vi "to table.vi"(8 "error in (no error)":errorcluster, 10 "variant":variant, 11 "Scaling editor node in":refnum<class "Scaling editor node.lvclass">) -> (0 "error out":errorcluster, 2 "table":string[][](array[string]), 3 "Scaling editor node out":refnum<class "Scaling editor node.lvclass">)   [LabVIEW 2013, in "Scaling editor node.lvclass"]
uses:
  Scaling editor node.lvclass
  module/configuration/Scaling configuration.lvclass
  <vilib>/NI/Module Execution Interface/Engine Configuration/engine configuration.lvclass
  Scaling editor node.lvclass/Scaling editor node.ctl
  <vilib>/NI/Configuration Framework/serializable configuration/NISE_CEF_serializable configuration.lvclass/NISE_CEF_serializable configuration.ctl
  <vilib>/NI/Tag Bus/tag/tag descriptor.lvclass/tag descriptor.ctl
  <vilib>/Utility/LVClass/Get LV Class Name.vi
  <vilib>/NI/Configuration Framework/error generator/NISE_error generator.vi
  <vilib>/NI/Tag Bus/tag/tag descriptor.lvclass
  <vilib>/NI/Configuration Framework/serializable configuration/NISE_CEF_serializable configuration.lvclass
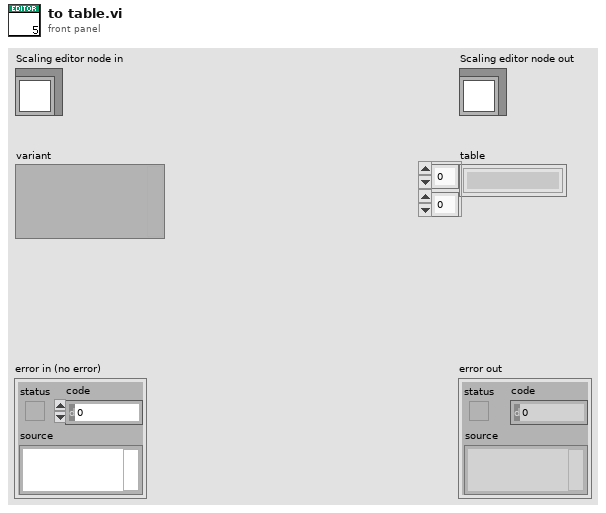
[diagram p1: front panel]
types:
  T1 = typedef "Scaling configuration.lvclass/scale data types.ctl" = enum16{"Double", "Single", "I64", "I32", "I16", "I8", "U64", "U32", "U16", "U8"}
  T2 = cluster{"input channel":refnum<class "TBM channel.lvclass">, "output channel":refnum<class "TBM channel.lvclass">, "input data type":T1, "output data type":T1}[]
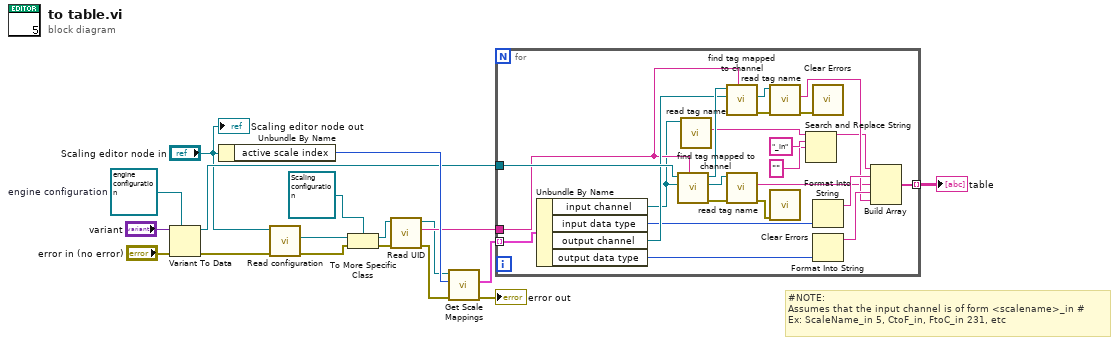
[diagram p0: block diagram]
diagram:
  w14 = refnum<class "engine configuration.lvclass"> refnum  # engine configuration
  # "#NOTE:\nAssumes that the input channel is of form <scalename>_in #\nEx: ScaleName_in 5, CtoF_in, FtoC_in 231, etc"
  n1 = Variant To Data(error in="error in (no error)", type=w14, Variant="variant") -> (data=w12:refnum<class "engine configuration.lvclass">, error out=w10:errorcluster)
  n2 = Unbundle By Name("Scaling editor node in") -> ("active scale index"=w15:i32)
  n3 = call-dynamic "Read configuration.vi"("error in"=w10, "Scaling editor node in"="Scaling editor node in") -> ("error out"=w16:errorcluster, "configuration"=w17:refnum<class "NISE_CEF_serializable configuration.lvclass">)  [unwired: 7 in, 1 out]
  n4 = To More Specific Class(target class=refnum<class "Scaling configuration.lvclass"> refnum ("Scaling configuration"), reference=w17, error in=w16) -> (specific class reference=w7:refnum<class "Scaling configuration.lvclass">, error out=w4:errorcluster)
  n5 = call <vilib>:"Read UID.vi"("error in"=w4, "configuration in"=w7) -> ("error out"=w3:errorcluster, "instance id"=w6:string, "configuration out"=w5:refnum<class "Scaling configuration.lvclass">)  [unwired: 7 in]
  n6 = call "Get Scale Mappings.vi"("error in (no error)"=w3, "index"=w15, "Scaling configuration in"=w5) -> ("error out"=→"error out":errorcluster, "mappings"=w9:T2)  [unwired: 6 in, 1 out]
  n7 = for {
    tunnel: w9 -> [w41] mode=indexing
    tunnel: w12 -> [w40]
    tunnel: [w30] -> w8 mode=indexing
    tunnel: w6 -> [w29]
    n8 = Unbundle By Name(w41) -> ("input channel"=w20:refnum<class "TBM channel.lvclass">, "input data type"=w32:T1, "output channel"=w33:refnum<class "TBM channel.lvclass">, "output data type"=w31:T1)
    n9 = call <vilib>:"find tag mapped to channel.vi"("owner"=w29, "channel"=w20, "engine configuration in"=w40) -> ("error out"=w38:errorcluster, "tag"=w39:refnum<class "tag descriptor.lvclass">, "engine configuration out"=w34:refnum<class "engine configuration.lvclass">)  [unwired: 6 in]
    n10 = call <vilib>:"read tag name.vi"("system tag in"=w20) -> ("name"=w19:string)  [unwired: 8 in, 2 out]
    n11 = call <vilib>:"find tag mapped to channel.vi"("owner"=w29, "channel"=w33, "engine configuration in"=w34) -> ("error out"=w35:errorcluster, "tag"=w28:refnum<class "tag descriptor.lvclass">)  [unwired: 6 in, 1 out]
    n12 = call <vilib>:"read tag name.vi"("error in"=w38, "system tag in"=w39) -> ("error out"=w37:errorcluster, "name"=w24:string)  [unwired: 7 in, 1 out]
    n13 = call <vilib>:"read tag name.vi"("error in"=w35, "system tag in"=w28) -> ("error out"=w36:errorcluster, "name"=w25:string)  [unwired: 7 in, 1 out]
    n14 = call <vilib>:"Clear Errors.vi"("error in (no error)"=w37) -> ()  [unwired: 6 in, 1 out]
    n15 = Search and Replace String(input string=w19, search string="_in", replace string="" ("replace string (\"\")")) -> (result string=w21:string)  [unwired: 5 in, 3 out]
    n16 = call <vilib>:"Clear Errors.vi"("error in (no error)"=w36) -> ()  [unwired: 6 in, 1 out]
    n17 = Format Into String(w32) -> (resulting string=w27:string)  [unwired: 3 in, 1 out]
    n18 = Format Into String(w31) -> (resulting string=w26:string)  [unwired: 3 in, 1 out]
    n19 = Build Array(w21, w27, w24, w26, w25) -> (w30:string[])
  }
  "table" <- w8
  "Scaling editor node out" <- "Scaling editor node in"
